vi "Unit Test Preserve wired serialized data (Same) False.vi"() -> ()   [LabVIEW 2019, in "Sports Unit Tests.lvclass"]
uses:
  Sports Unit Tests.lvclass
  <userlib>/Blue Origin/BlueSerialization/BlueSerializer/DeserializeOptions.ctl
  <userlib>/Blue Origin/BlueSerialization/BlueSerializer/DeserializeSlicingOptions.ctl
  <userlib>/Blue Origin/BlueSerialization/BlueSerializer/DeserializeMutationOptions.ctl
  <userlib>/Blue Origin/BlueSerialization/BlueSerializer/DeserializePreservationOptions.ctl
  <userlib>/Blue Origin/BlueSerialization/BlueSerializer/PreserveNonWiredDataOption.ctl
  Classes/Adam Sandler/Adam Sandler.lvclass
  C:/DSCE code/Serialization/blueserializationdemo/Test/Sports/Classes/Human/Human.lvclass
  C:/DSCE code/Serialization/blueserializationdemo/Test/Sports/Classes/Sports Player/Sports Player.lvclass
  C:/DSCE code/Serialization/blueserializationdemo/Test/Sports/Classes/Golf Player/Golf Player.lvclass
  Classes/Human/Human.lvclass/Human.ctl
  Classes/Sports Player/Sports Player.lvclass/Sports Player.ctl
  Classes/Golf Player/Golf Player.lvclass/Golf Player.ctl
  Classes/Adam Sandler/Adam Sandler.lvclass/Adam Sandler.ctl
  Classes/Human/Write Age (years).vi
  Classes/Human/Write alive_.vi
  Classes/Human/Write Height (ft).vi
  Classes/Human/Write Name.vi
  Classes/Sports Player/Write Earnings (dollars).vi
  Classes/Sports Player/Write Professional_.vi
  Classes/Sports Player/Write Sponsor.vi
  Classes/Golf Player/Write # holes in one.vi
  Classes/Golf Player/Write League.vi
  Classes/Golf Player/Write longest drive (ft).vi
  Classes/Adam Sandler/Write Movie Name.vi
  Classes/Adam Sandler/Write Private number.vi
  Classes/Adam Sandler/Write Secret phrase.vi
  Classes/Adam Sandler/Read Secret phrase.vi
  Classes/Human/Read Name.vi
  <vilib>/Utility/error.llb/Clear Errors.vi
  <vilib>/addons/_JKI Toolkits/Caraya/classes/Test/Define Test.vi
  <vilib>/addons/_JKI Toolkits/Caraya/classes/Assert/Assert Equal Value_Variant.vi
  <vilib>/addons/_JKI Toolkits/Caraya/classes/Assert/Assert Not Error.vi
  <userlib>/Blue Origin/BlueSerialization/BlueSerializer/BlueSerializer.lvclass
  <vilib>/addons/_JKI Toolkits/Caraya/classes/Assert/Assert.lvclass
  C:/Program Files (x86)/National Instruments/LabVIEW 2019/user.lib/Blue Origin/BlueSerialization/BlueSerializable/BlueSerializable.lvclass
panel:
  out "Table":string[][](table)=[["{\r  \"Class\":[\"Adam Sandler.lvclass\",\"Golf Player.lvclass\",\"Sports Player.lvclass\",\"Human.lvclass\",\"Root\"],\r  \"Version\":[\"2.0.0.3\",\"2.0.0.3\",\"2.0.0.3\",\"2.0.0.3\",\"2.0.0.0\"],\r  \"Human.lvclass\":{\r    \"alive?\":true,\r    \"Age (years)\":31,\r    \"Height (ft)\":6\r  },\r  \"Sports Player.lvclass\":{\r    \"Professional?\":true,\r    \"Earnings (dollars)\":1000000,\r    \"Sponsor\":\"Monster Energy\"\r  },\r  \"Golf Player.lvclass\":{\r    \"League\":\"Happy Gilmore league\",\r    \"# holes in one\":999,\r    \"longest drive (ft)\":88888\r  },\r  \"Adam Sandler.lvclass\":{\"Movie Name\":\"Happy Gilmore\"}\r}", "{\r  \"Class\":[\"Adam Sandler.lvclass\",\"Golf Player.lvclass\",\"Sports Player.lvclass\",\"Human.lvclass\",\"Root\"],\r  \"Version\":[\"2.0.0.3\",\"2.0.0.3\",\"2.0.0.3\",\"2.0.0.3\",\"2.0.0.0\"],\r  \"Human.lvclass\":{\r    \"alive?\":true,\r    \"Age (years)\":31,\r    \"Name\":\"Happy Gilmore\",\r    \"Height (ft)\":6\r  },\r  \"Sports Player.lvclass\":{\r    \"Professional?\":true,\r    \"Earnings (dollars)\":1000000,\r    \"Sponsor\":\"Monster Energy\"\r  },\r  \"Golf Player.lvclass\":{\r    \"League\":\"Happy Gilmore league\",\r    \"# holes in one\":999,\r    \"longest drive (ft)\":88888\r  },\r  \"Adam Sandler.lvclass\":{\"Movie Name\":\"Happy Gilmore\"}\r}", "Status: FALSE\ncode: 0\n", "BlueJSONTextSerializer.lvlib:BlueJSONTextSerializer.lvclass"], ["Class = [\"Adam Sandler.lvclass\", \"Golf Player.lvclass\", \"Sports Player.lvclass\", \"Human.lvclass\", \"Root\"]\r\nVersion = [\"2.0.0.3\", \"2.0.0.3\", \"2.0.0.3\", \"2.0.0.3\", \"2.0.0.0\"]\r\n\n[\"Human.lvclass\"]\n\"alive?\" = true\r\n\"Age (years)\" = 31\r\n\"Height (ft)\" = 6.0\r\n\n[\"Sports Player.lvclass\"]\n\"Professional?\" = true\r\n\"Earnings (dollars)\" = 1000000.0\r\nSponsor = \"Monster Energy\"\r\n\n[\"Golf Player.lvclass\"]\nLeague = \"Happy Gilmore league\"\r\n\"# holes in one\" = 999\r\n\"longest drive (ft)\" = 88888.0\r\n\n[\"Adam Sandler.lvclass\"]\n\"Movie Name\" = \"Happy Gilmore\"\r\n", "Class = [\"Adam Sandler.lvclass\", \"Golf Player.lvclass\", \"Sports Player.lvclass\", \"Human.lvclass\", \"Root\"]\r\nVersion = [\"2.0.0.3\", \"2.0.0.3\", \"2.0.0.3\", \"2.0.0.3\", \"2.0.0.0\"]\r\n\n[\"Human.lvclass\"]\n\"alive?\" = true\r\n\"Age (years)\" = 31\r\nName = \"Happy Gilmore\"\r\n\"Height (ft)\" = 6.0\r\n\n[\"Sports Player.lvclass\"]\n\"Professional?\" = true\r\n\"Earnings (dollars)\" = 1000000.0\r\nSponsor = \"Monster Energy\"\r\n\n[\"Golf Player.lvclass\"]\nLeague = \"Happy Gilmore league\"\r\n\"# holes in one\" = 999\r\n\"longest drive (ft)\" = 88888.0\r\n\n[\"Adam Sandler.lvclass\"]\n\"Movie Name\" = \"Happy Gilmore\"\r\n", "Status: FALSE\ncode: 0\n", "BlueTOMLSerializer.lvlib:BlueTOMLSerializer.lvclass"]]
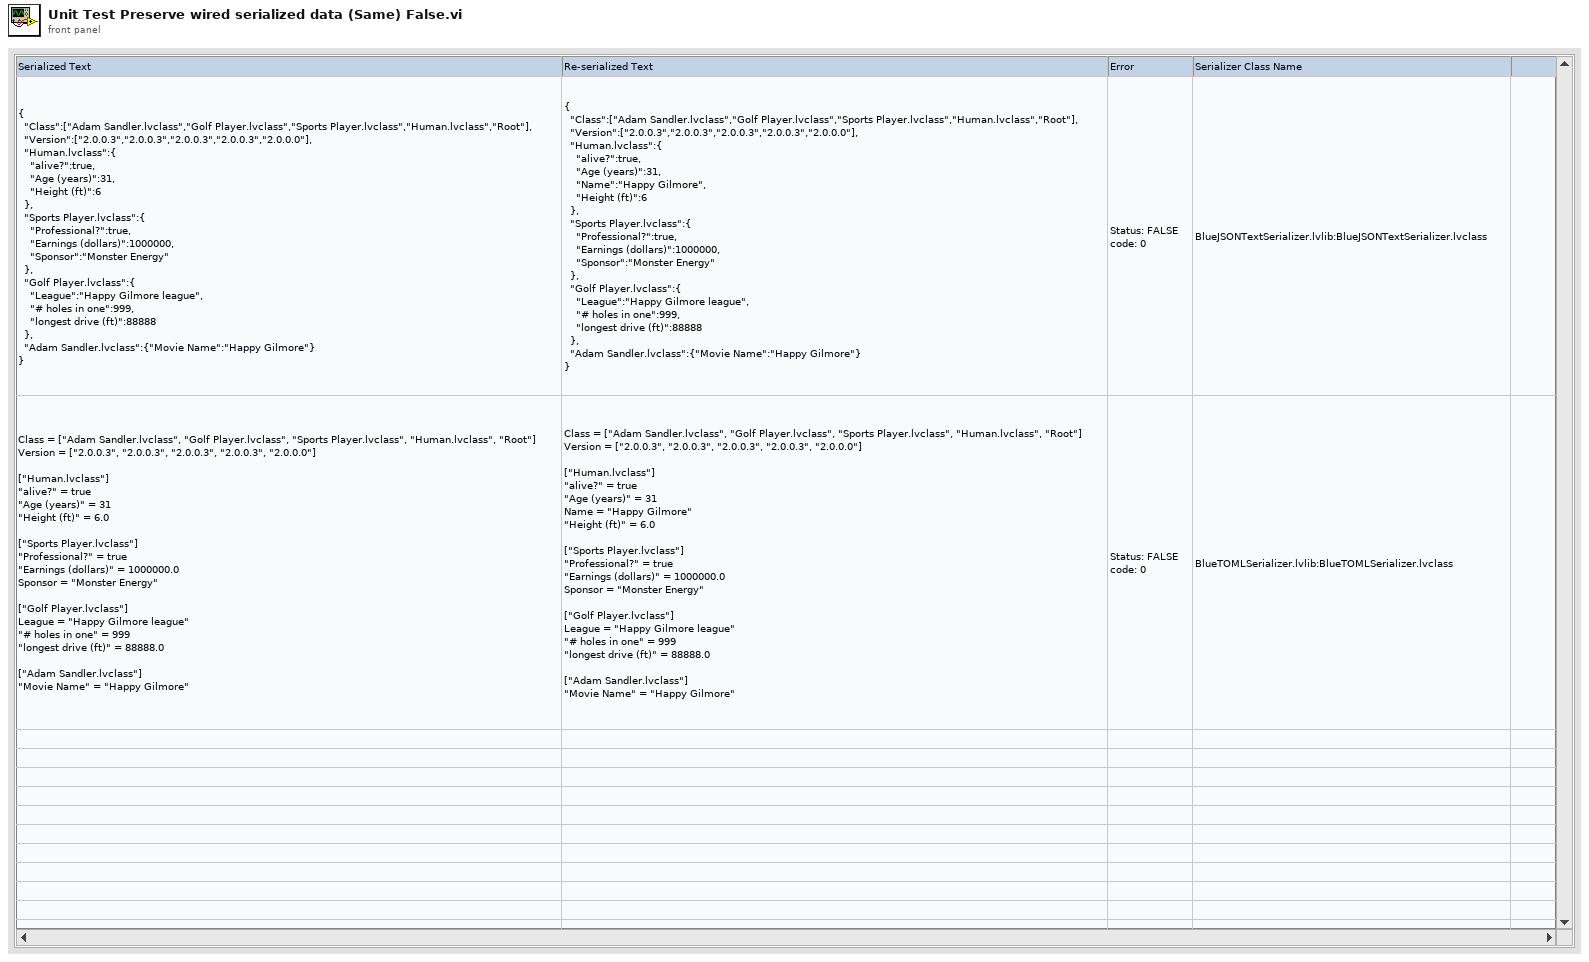
[diagram p1: front panel]
types:
  T1 = typedef "BlueSerialization.lvlib/BlueSerializer.lvclass/DeserializeOptions.ctl" = cluster{"deserialize non-BlueSerializable objects from hex?":bool, "expand objects on type conflict?":bool, "Slicing":T2, "Mutation Options":T3, "Preservation Options":T4}
  T2 = typedef "BlueSerialization.lvlib/BlueSerializer.lvclass/DeserializeSlicingOptions.ctl" = cluster{"slice flattened object data on error?":bool, "sliceable class names":string[]}
  T3 = typedef "BlueSerialization.lvlib/BlueSerializer.lvclass/DeserializeMutationOptions.ctl" = cluster{"error on inserted parent levels?":bool, "\terror on obsolete parent levels?":bool}
  T4 = typedef "BlueSerialization.lvlib/BlueSerializer.lvclass/DeserializePreservationOptions.ctl" = cluster{"Preserve wired serialized data?":bool, "Preserve wired non-serialized data":T5}
  T5 = typedef "BlueSerialization.lvlib/BlueSerializer.lvclass/PreserveNonWiredDataOption.ctl" = enum16{"Don't preserve", "Preserve (error on less-specific wired types)", "Preserve (except on less-specific wired types)"}
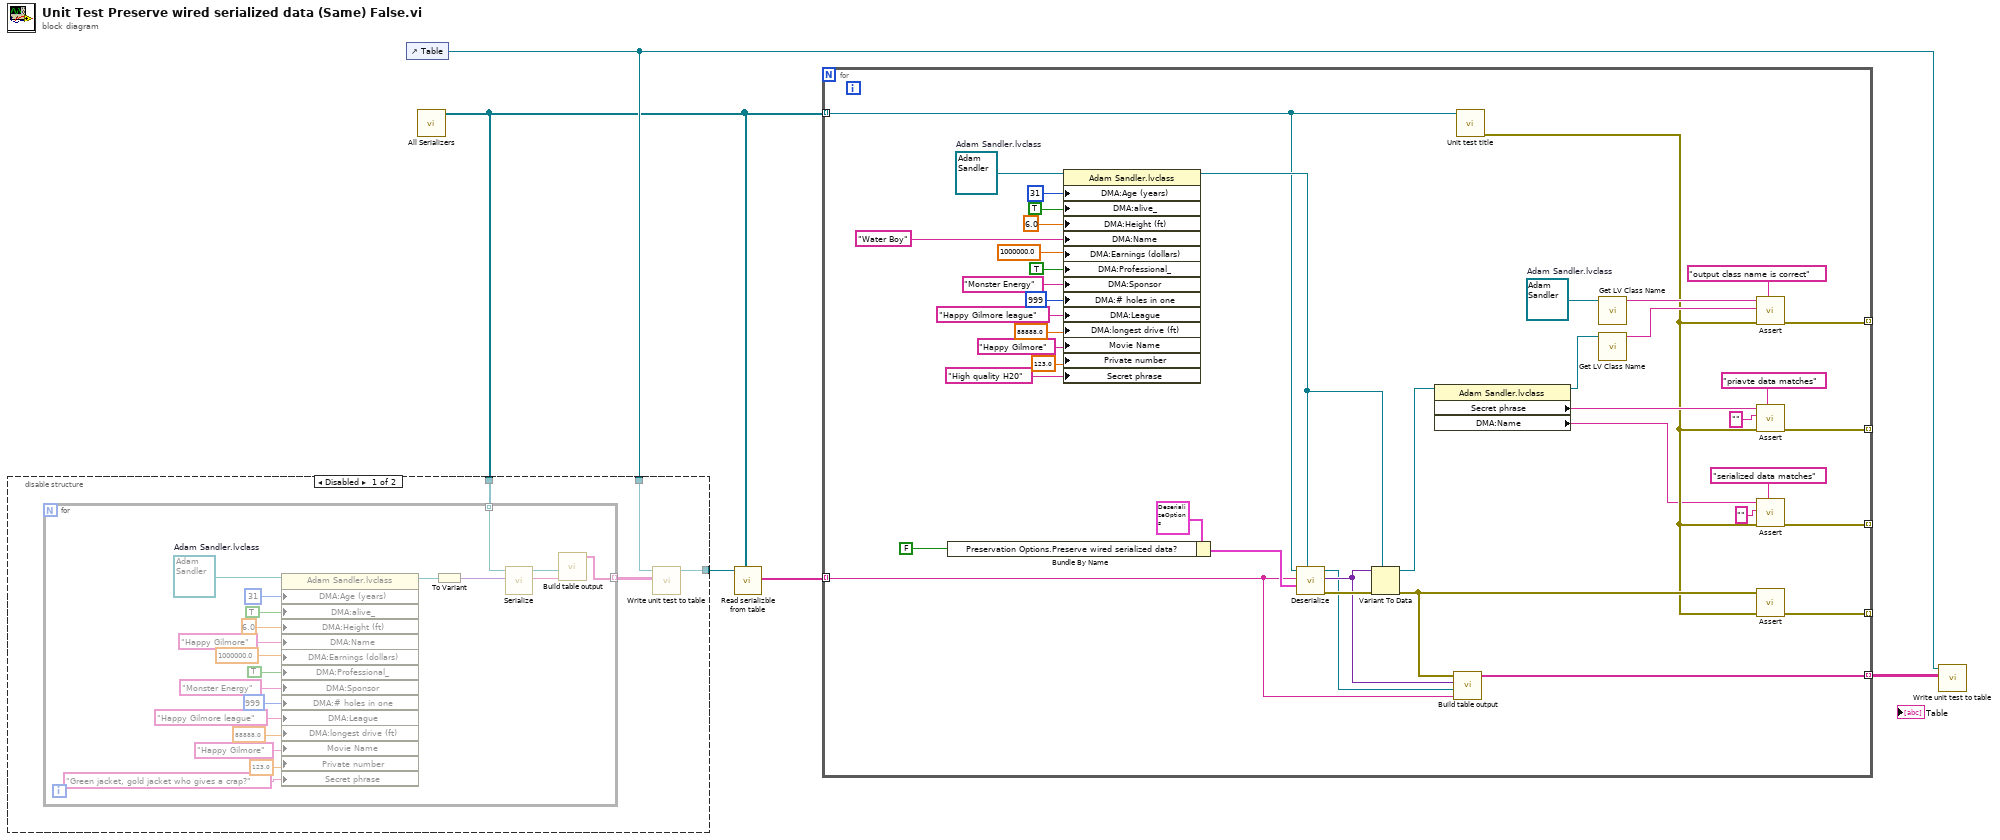
[diagram p0: block diagram]
diagram:
  n1 = control-ref of="Table"() -> (w4:refnum<vi>)
  n2 = call "All Serializers.vi"() -> ("All serializers"=w2:refnum<class "BlueSerializer.lvclass">[])  [unwired: 11 in]
  n3 = disable-structure shown="Disabled" {
    disable-tunnel: w4 -> [w8 w30]
    disable-tunnel: [w7 w30] -> w3
    disable-tunnel: w2 -> [w6 _]
    frame Disabled {
      n4 = for {
        tunnel: w6 -> [w28] mode=indexing
        tunnel: [w25] -> w9 mode=indexing
        w18 = refnum<class "Adam Sandler.lvclass"> refnum  # Adam Sandler.lvclass
        n5 = property on="Property Node" class="Adam Sandler.lvclass"(reference=w18, "DMA:Age (years)"=u16 31 ("Age (years)"), "DMA:alive_"=TRUE ("alive_"), "DMA:Height (ft)"=6.0 ("Height (ft)"), "DMA:Name"="Happy Gilmore" ("Name"), "DMA:Earnings (dollars)"=1000000.0 ("Earnings (dollars)"), "DMA:Professional_"=TRUE ("Professional_"), "DMA:Sponsor"="Monster Energy" ("Sponsor"), "DMA:# holes in one"=999 ("# holes in one"), "DMA:League"="Happy Gilmore league" ("League"), "DMA:longest drive (ft)"=88888.0 ("longest drive (ft)"), "Movie Name"="Happy Gilmore", "Private number"=123.0, "Secret phrase"="Green jacket, gold jacket who gives a crap?") -> (reference out=w10:refnum<class "Adam Sandler.lvclass">)  [unwired: 1 in, 1 out]
        n6 = To Variant(anything=w10) -> (Variant=w29:variant)
        n7 = call <userlib>:"Serialize.vi"("Anything"=w29, "BlueSerializer in"=w28) -> ("Serialized Text"=w27:string, "BlueSerializer out"=w26:refnum<class "BlueSerializer.lvclass">)  [unwired: 7 in, 1 out]
        n8 = call "Build table output.vi"("serialized text"=w27, "BlueSerializer in"=w26) -> ("table output"=w25:string[])  [unwired: 9 in]
      }
      n9 = call "Write unit test to table.vi"("Table"=w9, "Table ref in"=w8) -> ("Table ref out"=w7:refnum<vi>)  [unwired: 9 in]
    }
    frame Enabled {
    }
  }
  n10 = call "Read serializble from table.vi"("serializers"=w2, "Table ref in"=w3) -> ("serializable texts"=w1:string[])  [unwired: 7 in, 2 out]
  n11 = for {
    tunnel: w2 -> [w32] mode=indexing
    tunnel: [w68] -> _ mode=indexing
    tunnel: [w67] -> _ mode=indexing
    tunnel: [w63] -> w5 mode=indexing
    tunnel: [w57] -> _ mode=indexing
    tunnel: [w38] -> _ mode=indexing
    tunnel: w1 -> [w33] mode=indexing
    w48 = refnum<class "Adam Sandler.lvclass"> refnum  # Adam Sandler.lvclass
    w62 = refnum<class "Adam Sandler.lvclass"> refnum  # Adam Sandler.lvclass
    n12 = Bundle By Name(cluster=T1 {"deserialize non-BlueSerializable objects from hex?"=FALSE, "expand objects on type conflict?"=FALSE, "Slicing"={"slice flattened object data on error?"=FALSE, "sliceable class names"=[]}, "Mutation Options"={"error on inserted parent levels?"=FALSE, "\terror on obsolete parent levels?"=FALSE}, "Preservation Options"={"Preserve wired serialized data?"=FALSE, "Preserve wired non-serialized data"=enum."Don't preserve"}} ("Deserialize Options"), "Preservation Options.Preserve wired serialized data?"=FALSE ("Allow class expansion?")) -> (w54:T1)
    n13 = property on="Property Node" class="Adam Sandler.lvclass"(reference=w48, "DMA:Age (years)"=u16 31 ("Age (years)"), "DMA:alive_"=TRUE ("alive_"), "DMA:Height (ft)"=6.0 ("Height (ft)"), "DMA:Name"="Water Boy" ("Name"), "DMA:Earnings (dollars)"=1000000.0 ("Earnings (dollars)"), "DMA:Professional_"=TRUE ("Professional_"), "DMA:Sponsor"="Monster Energy" ("Sponsor"), "DMA:# holes in one"=999 ("# holes in one"), "DMA:League"="Happy Gilmore league" ("League"), "DMA:longest drive (ft)"=88888.0 ("longest drive (ft)"), "Movie Name"="Happy Gilmore", "Private number"=123.0, "Secret phrase"="High quality H20") -> (reference out=w41:refnum<class "Adam Sandler.lvclass">)  [unwired: 1 in, 1 out]
    n14 = call <userlib>:"Deserialize.vi"("Anything"=w41, "Deserialize Options"=w54, "Serialized Text"=w33, "BlueSerializer in"=w32) -> ("error out"=w72:errorcluster, "Variant"=w65:variant, "BlueSerializer out"=w64:refnum<class "BlueSerializer.lvclass">)  [unwired: 5 in]
    n15 = Variant To Data(error in=w72, type=w41, Variant=w65) -> (data=w60:refnum<class "Adam Sandler.lvclass">, error out=w66:errorcluster)
    n16 = property class="Adam Sandler.lvclass"(reference=w60) -> (reference out=w59:refnum<class "Adam Sandler.lvclass">, "Secret phrase"=w58:string, "DMA:Name"=w35:string)  [unwired: 1 in, 1 out]
    n17 = call "Build table output.vi"("serialized text"=w33, "BlueSerializer in"=w64, "deserialized variant"=w65, "variant to data error"=w66) -> ("table output"=w63:string[])  [unwired: 7 in]
    n18 = call "Unit test title.vi"("serializer"=w32) -> ("error out"=w36:errorcluster)  [unwired: 9 in, 1 out]
    n19 = call <vilib>:"Get LV Class Name.vi"("object"=w62) -> ("class name"=w71:string)  [unwired: 9 in, 1 out]
    n20 = call <vilib>:"Get LV Class Name.vi"("object"=w59) -> ("class name"=w70:string)  [unwired: 9 in, 1 out]
    n21 = call-poly <vilib>:"Assert.vi"("Label"="output class name is correct", "error in (no error)"=w36, "Y"=w70, "X"=w71) -> ("error out"=w67:errorcluster)  [unwired: 7 in]
    n22 = call-poly <vilib>:"Assert.vi"("Label"="priavte data matches", "error in (no error)"=w36, "Y"="" ("Secret phrase"), "X"=w58) -> ("error out"=w57:errorcluster)  [unwired: 7 in]
    n23 = call-poly <vilib>:"Assert.vi"("Label"="serialized data matches", "error in (no error)"=w36, "Y"="" ("Name"), "X"=w35) -> ("error out"=w38:errorcluster)  [unwired: 7 in]
    n24 = call-poly <vilib>:"Assert.vi"("error in (no error)"=w36, "Not Error?"=w66) -> ("error out"=w68:errorcluster)  [unwired: 9 in]
  }
  n25 = call "Write unit test to table.vi"("Table"=w5, "Table ref in"=w4) -> ()  [unwired: 9 in, 1 out]
